vi "VISA.vi"() -> ()   [LabVIEW 2017]
uses:
  <vilib>/Instr/_visa.llb/VISA Configure Serial Port (Instr).vi
panel:
  in  "Stop Button":bool
  out "Read Buffer":string
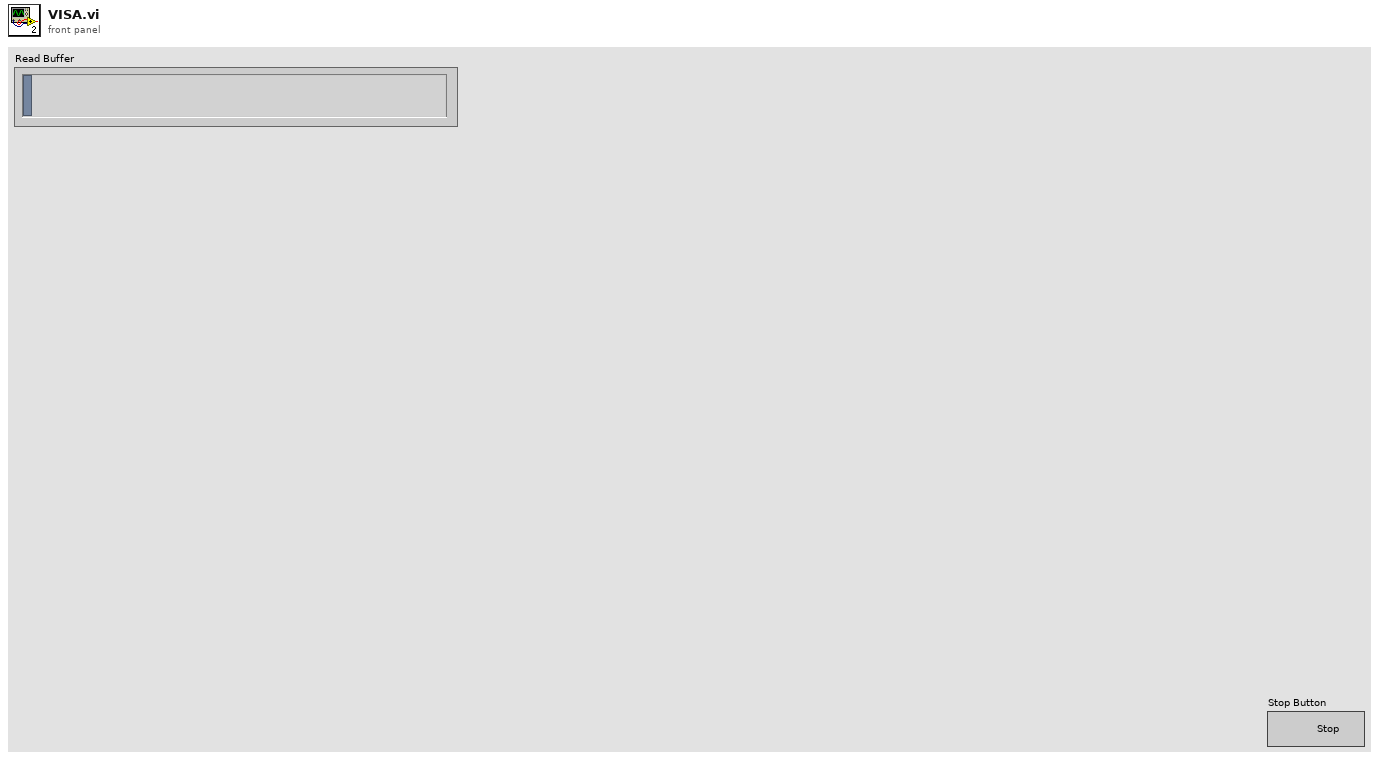
[diagram p1: front panel]
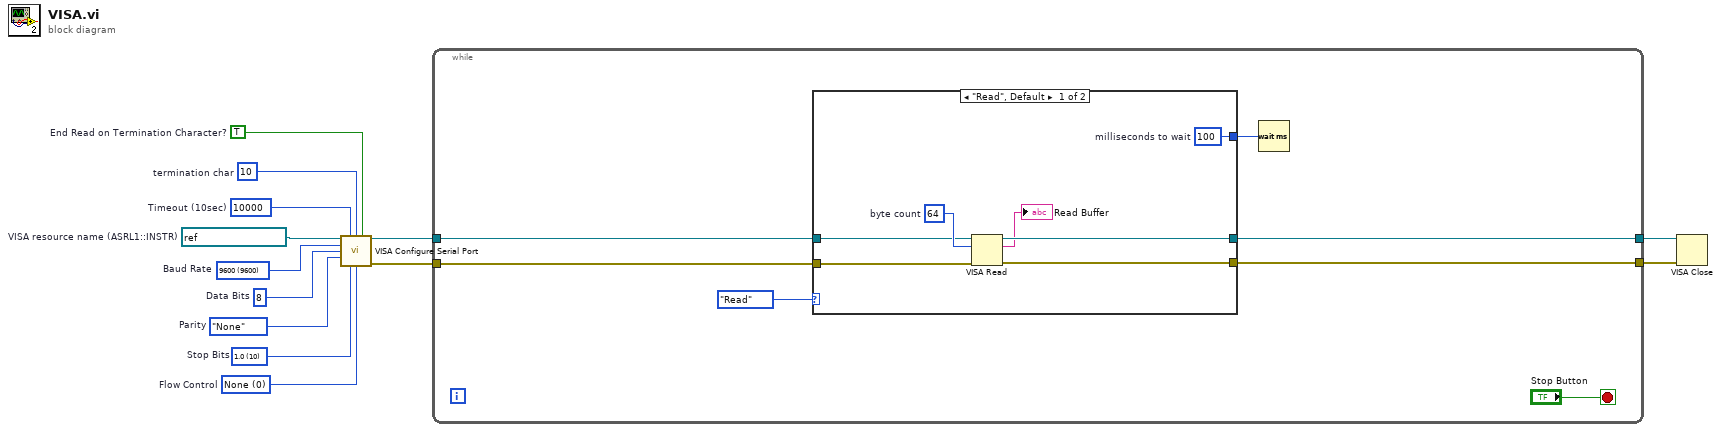
[diagram p0: block diagram]
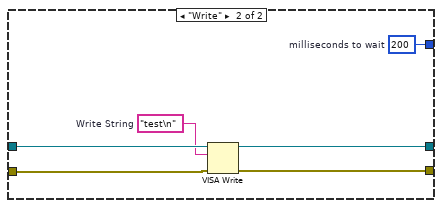
[diagram p2: hidden frame]
diagram:
  w1 = 10  # termination char
  w8 = u16 10 items=["1.0"=10, "1.5"=15, "2.0"=20]  # Stop Bits
  w9 = enum16{"None", "Odd", "Even", "Mark", "Space"}."None"  # Parity
  w10 = u16 8  # Data Bits
  w11 = u32 9600 items=["75"=75, "110"=110, "134"=134, "150"=150, "300"=300, "600"=600, "1200"=1200, "1800"=1800, "2400"=2400, "4800"=4800, "7200"=7200, "9600"=9600, "14400"=14400, "19200"=19200, "28800"=28800, "38400"=38400, "56000"=56000, "57600"=57600, "115200"=115200, "128000"=128000, "230400"=230400]  # Baud Rate
  w13 = refnum<visa-resource-name> "ASRL1::INSTR"  # VISA resource name (ASRL1::INSTR)
  w12 = TRUE  # End Read on Termination Character?
  w6 = u32 10000  # Timeout (10sec)
  w7 = u16 0 items=["None"=0, "XON/XOFF"=1, "RTS/CTS"=2, "DTR/DSR"=4]  # Flow Control
  n1 = call-poly "VISA Configure Serial Port"("VISA resource name"=w13, "timeout (10sec)"=w6, "termination char\n(0xA = '\\n' = LF)"=w1, "Enable Termination\nChar (T)"=w12, "baud rate (9600)"=w11, "data bits (8)"=w10, "parity (0:none)"=w9, "stop bits (10: 1 bit)"=w8, "flow control (0:none)"=w7) -> ("VISA resource name out"=w5:refnum<visa-resource-name>, "error out"=w4:errorcluster)  [unwired: 1 in, 4 out]
  n2 = while {
    tunnel: w5 -> [w19]
    tunnel: w4 -> [w18]
    tunnel: [w17] -> w3
    tunnel: [w16] -> w2
    stop <- "Stop Button" stop-if-true
    n3 = case shown="\"Read\", Default" enum16{"Read", "Write"}."Read" ("Enum") {
      tunnel: w19 -> [w22 w33]
      tunnel: [w26 w32] -> w17
      tunnel: [w27 w31] -> w16
      tunnel: [w24 w29] -> w20
      tunnel: w18 -> [w21 w28]
      frame "Read", Default {
        w23 = u32 64  # byte count
        w24 = u32 100  # milliseconds to wait
        n4 = VISA Read(VISA resource name=w22, byte count=w23, error in (no error)=w21) -> (VISA resource name out=w26:refnum<visa-resource-name>, read buffer=→"Read Buffer":string, error out=w27:errorcluster)  [unwired: 1 out]
      }
      frame "Write" {
        w29 = u32 200  # milliseconds to wait
        w30 = "test\n"  # Write String
        n5 = VISA Write(VISA resource name=w33, write buffer=w30, error in (no error)=w28) -> (VISA resource name out=w32:refnum<visa-resource-name>, error out=w31:errorcluster)  [unwired: 1 out]
      }
    }
    n6 = Wait (ms)(milliseconds to wait=w20) -> ()  [unwired: 1 out]
  }
  n7 = VISA Close(VISA resource name=w3, error in (no error)=w2) -> ()  [unwired: 1 out]
